vi "Get Instruments Required From Test Step.vi"(8 "error in (no error)":errorcluster, 9 "Instruments on Station":T1[](array[typedef]), 11 "Test_ID (\"\")":string) -> (0 "error out":errorcluster, 1 "Required Instruments":T1[](array[typedef]), 2 "Instrument Types":string[](array[string]))   [LabVIEW 2011]
uses:
  server/database/Stations/Instruments/Instrument Record.ctl
  Test Function.ctl
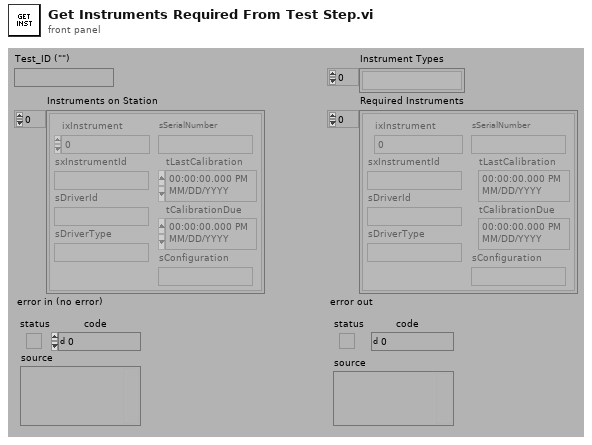
[diagram p1: front panel]
types:
  T1 = typedef "Instrument Record.ctl" = cluster{"ixInstrument":i32, "sxInstrumentId":string, "sDriverId":string, "sDriverType":string, "sSerialNumber":string, "tLastCalibration":timestamp, "tCalibrationDue":timestamp, "sConfiguration":string}
  T2 = typedef "Test Function.ctl" = enum16{"Test Config", "Test Storage", "Test Pre-Process", "Unflatten Test Parameters", "Flatten Test Parameters"}
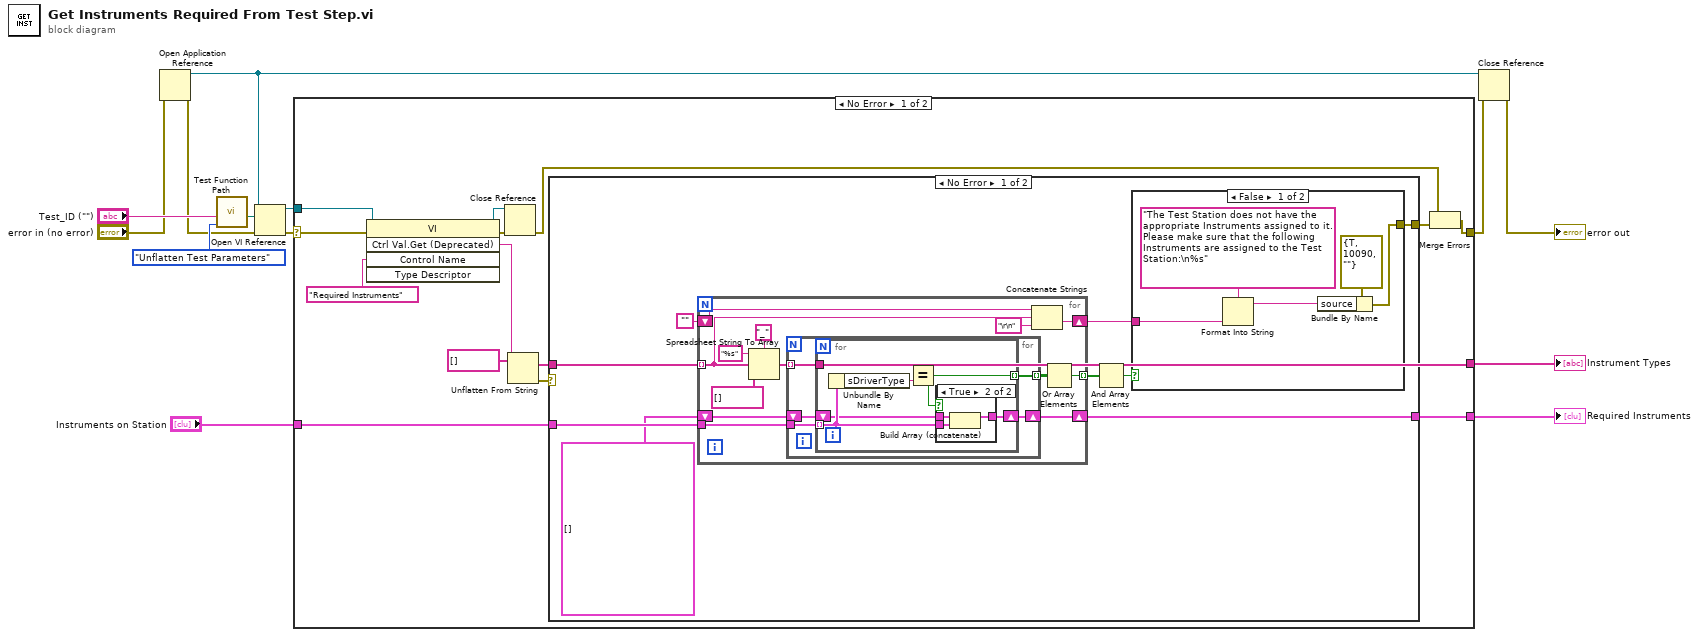
[diagram p0: block diagram]
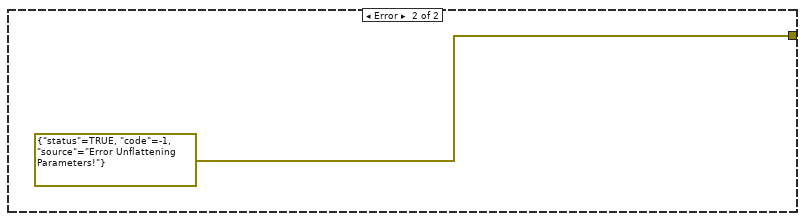
[diagram p4: hidden frame]
diagram:
  n1 = Open Application Reference(8:"error in (no error)") -> (0:w2:errorcluster, 3:w1:refnum<vi>)  [unwired: 3 in]
  n2 = call "Test Function Path.vi"("Object Type (Test Config)"=Test_Function."Unflatten Test Parameters", "Object Name (\"\")"="Test_ID (\"\")") -> ("Object Path"=w9:path)  [unwired: 1 in, 8 out]
  n3 = Open VI Reference(application reference (local)=w1, vi path=w9, error in (no error)=w2) -> (vi reference=w11:refnum<vi>, error out=w12:errorcluster)  [unwired: 1 in, 2 out]
  n4 = case shown="No Error" w12 {
    selector: w12 -> [w22 w71]
    tunnel: w11 -> [w23 _]
    tunnel: "Instruments on Station" -> [w19 _]
    tunnel: [w18 w71] -> w4
    tunnel: [w16 _] -> w7
    tunnel: [w15 _] -> w6
    frame No Error {
      n5 = invoke class="VI" method="Ctrl Val.Get (Deprecated)"(reference=w23, error in=w22, "Control Name"="Required Instruments") -> (reference out=w24:refnum<vi>, error out=w25:errorcluster, "Get Control Value"=w26:string)  [unwired: 2 in, 2 out]
      n6 = Close Reference(reference=w24, error in (no error)=w25) -> (error out=w14:errorcluster)
      n7 = Unflatten From String(type=string[] [], binary string=w26) -> (value=w15:string[], error out=w17:errorcluster)  [unwired: 1 in, 3 out]
      n8 = case shown="No Error" w17 {
        tunnel: [w32 errorcluster {"status"=TRUE, "code"=-1, "source"="Error Unflattening Parameters!"} ("f")] -> w20
        tunnel: w15 -> [w35 _]
        tunnel: w19 -> [w34 _]
        tunnel: [w29 _] -> w16
        frame No Error {
          n9 = for {
            tunnel: w34 -> [w54]
            tunnel: w35 -> [w47] mode=indexing
            tunnel: [w44] -> w36 mode=indexing
            shift-right: [w51] -> w29
            shift-left: T1[] [] -> [w52]
            shift-right: [w42] -> w31
            shift-left: "" -> [w43]
            n10 = Spreadsheet String To Array(delimiter (Tab)="_", format string="%s" ("delimiter (Tab)"), spreadsheet string=w47, array type (2D Dbl)=string[] []) -> (array=w46:string[])
            n11 = for {
              tunnel: w54 -> [w59]
              shift-right: [w57] -> w51
              shift-left: w52 -> [w58]
              tunnel: w46 -> [w56] mode=indexing
              tunnel: [w55] -> w45 mode=indexing
              n12 = for {
                tunnel: w59 -> [w63] mode=indexing
                tunnel: [w64] -> w55 mode=indexing
                shift-right: [w61] -> w57
                shift-left: w58 -> [w62]
                tunnel: w56 -> [w60]
                n13 = Unbundle By Name(w63) -> ("sDriverType"=w65:string)
                n14 = Equal?(x=w60, y=w65) -> (x = y?=w64:bool)
                n15 = case shown="True" w64 {
                  tunnel: w63 -> [_ w69]
                  tunnel: w62 -> [w66 w68]
                  tunnel: [w66 w67] -> w61
                  frame False {
                  }
                  frame True {
                    n16 = Build Array (concatenate)(w68, w69) -> (w67:T1[])
                  }
                }
              }
            }
            n17 = Concatenate Strings(w43, w47, "\r\n" ("string")) -> (w42:string)
            n18 = Or Array Elements(Boolean array=w45) -> (logical OR=w44:bool)
          }
          n19 = And Array Elements(Boolean array=w36) -> (logical AND=w33:bool)
          n20 = case shown="False" w33 {
            tunnel: [w38 _] -> w32
            tunnel: w31 -> [w37 _]
            frame False {
              n21 = Format Into String(format string="The Test Station does not have the appropriate Instruments assigned to it.  Please make sure that the following Instruments are assigned to the Test Station:\n%s" ("source"), w37) -> (resulting string=w39:string)  [unwired: 2 in, 1 out]
              n22 = Bundle By Name(cluster=errorcluster {"status"=TRUE, "code"=10090, "source"=""} ("f"), "source"=w39) -> (w38:errorcluster)
            }
            frame True {
            }
          }
        }
        frame Error {
        }
      }
      n23 = Merge Errors(w14, w20) -> (w18:errorcluster)
    }
    frame Error {
    }
  }
  "Required Instruments" <- w7
  "Instrument Types" <- w6
  n24 = Close Reference(reference=w1, error in (no error)=w4) -> (error out=→"error out":errorcluster)
